vi "Analog_input_ch1_Continuous.vi"() -> ()   [LabVIEW 2019]
uses:
  <vilib>/DAQmx/read.llb/DAQmx Read (Analog Wfm 1Chan NSamp).vi
  <vilib>/DAQmx/create/channels.llb/DAQmx Create Channel (AI-Voltage-Basic).vi
  <vilib>/DAQmx/configure/timing.llb/DAQmx Timing (Sample Clock).vi
  <vilib>/DAQmx/miscellaneous.llb/DAQmx Fill In Error Info.vi
  <vilib>/Waveform/WDTOps.llb/WDT Append Waveforms DBL.vi
  <vilib>/Waveform/WDTFileIO.llb/Export Waveform To Spreadsheet File.vi
panel:
  out "Numeric":i32
  in  "stop":bool
  out "Waveform Graph":waveform(dbl)(graph)
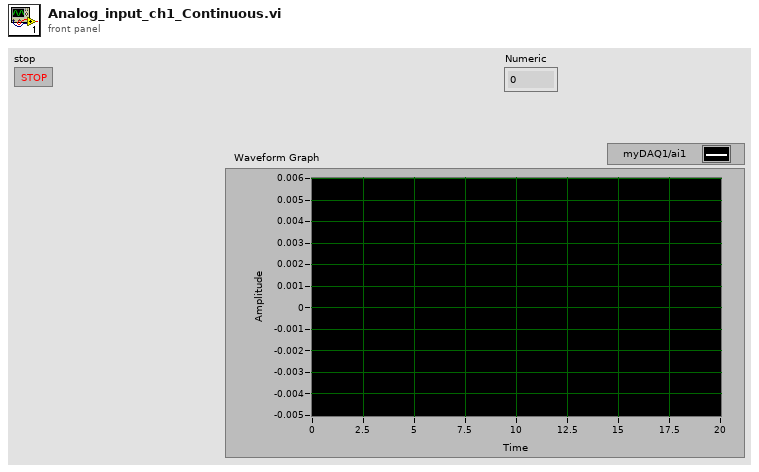
[diagram p1: front panel]
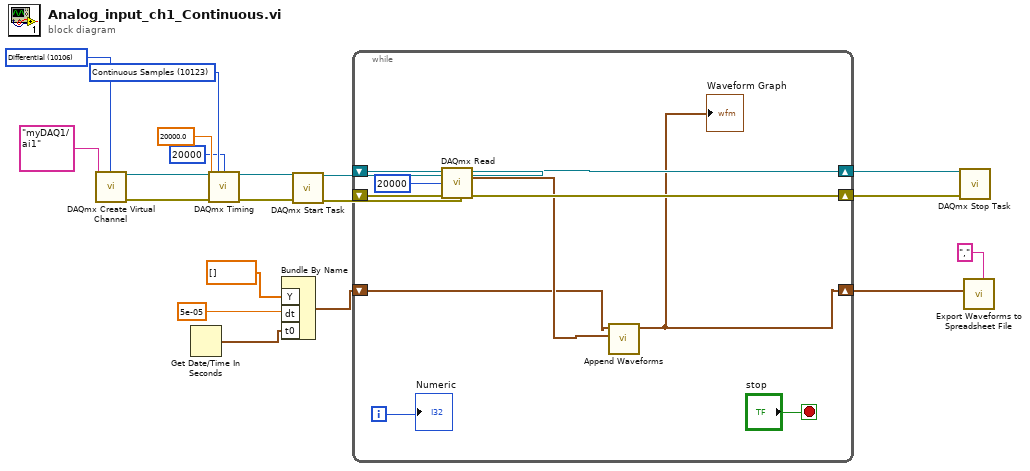
[diagram p0: block diagram]
diagram:
  w15 = 10123 items=["Finite Samples"=10178, "Continuous Samples"=10123, "Hardware Timed Single Point"=12522] ("sample mode")
  w18 = 10106 items=["Default"=-1, "RSE"=10083, "NRSE"=10078, "Differential"=10106, "Pseudodifferential"=12529] ("input terminal configuration")
  n1 = call-poly <vilib>:"DAQmx Create Virtual Channel.vi"("input terminal configuration"=w18, "physical channels"=tag "myDAQ1/ai1") -> ("task out"=w17:refnum<k21>, "error out"=w16:errorcluster)  [unwired: 12 in]
  n2 = Get Date/Time In Seconds() -> (seconds since 1Jan1904=w3:timestamp)
  n3 = call-poly <vilib>:"DAQmx Timing.vi"("task/channels in"=w17, "sample mode"=w15, "samples per channel"=20000, "rate"=20000.0, "error in"=w16) -> ("task out"=w8:refnum<k21>, "error out"=w7:errorcluster)  [unwired: 9 in]
  n4 = Bundle By Name("Y"=dbl[] [], "dt"=5e-05, "t0"=w3) -> (w2:waveform(dbl))  [unwired: 1 in]
  n5 = call <vilib>:"DAQmx Start Task.vi"("task/channels in"=w8, "error in"=w7) -> ("task out"=w12:refnum<k21>, "error out"=w11:errorcluster)  [unwired: 12 in]
  n6 = while {
    shift-right: [w26] -> w10
    shift-left: w12 -> [w29]
    shift-right: [w25] -> w9
    shift-left: w11 -> [w28]
    shift-right: [w20] -> w1
    shift-left: w2 -> [w21]
    i -> [w23]
    stop <- "stop" stop-if-true
    n7 = call-poly <vilib>:"DAQmx Read.vi"("task/channels in"=w29, "number of samples per channel"=20000, "error in"=w28) -> ("task out"=w26:refnum<k21>, "data"=w22:waveform(dbl), "error out"=w25:errorcluster)  [unwired: 10 in]
    n8 = call-poly <vilib>:"Append Waveforms.vi"("waveform B"=w22, "waveform A"=w21) -> ("waveform out"=w20:waveform(dbl))  [unwired: 8 in, 1 out]
    "Waveform Graph" <- w20
    "Numeric" <- w23
  }
  n9 = call <vilib>:"DAQmx Stop Task.vi"("task/channels in"=w10, "error in"=w9) -> ()  [unwired: 12 in, 2 out]
  n10 = call-poly <vilib>:"Export Waveforms to Spreadsheet File.vi"("delimiter (Tab)"=",", "waveform"=w1) -> ()  [unwired: 8 in, 2 out]
